vi "PathPlanner_PathFinder_ExtractPath.vi"(8 "error in (no error)":errorcluster) -> (0 "error out":errorcluster)   [LabVIEW 2019, in "PathPlanner24.lvlib"]
uses:
  PathPlanner24.lvlib
  TypeDef/PathPlannerFinderGridPosition.ctl
  PathPlanner_GridPosition_Get.vi
  PathPlanner_GridPosition_New.vi
  <vilib>/Rock Robotics/WPI/ThirdParty/JAS_Junk/TrajLib/Translation2d_Create.vi
  <vilib>/Rock Robotics/WPI/ThirdParty/JAS_Junk/TrajLib/Util_CalcDist.vi
  <vilib>/Rock Robotics/WPI/ThirdParty/JAS_Junk/TrajLib/Rotation2d_GetAngleCosSin.vi
  <vilib>/Rock Robotics/WPI/ThirdParty/JAS_Junk/TrajLib/Translation2d_GetXY.vi
  <vilib>/Rock Robotics/WPI/ThirdParty/JAS_Junk/TrajLib/Rotation2d_CreateXY.vi
  PathPlanner_PathFinder_Globals.vi
  <vilib>/Rock Robotics/WPI/ThirdParty/JAS_Junk/TrajLib/TypeDef/TRANSLATION2D.ctl
  <vilib>/Rock Robotics/WPI/ThirdParty/JAS_Junk/TrajLib/Trajectory_Library.lvlib
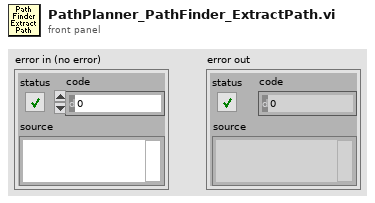
[diagram p1: front panel]
types:
  T1 = typedef "PathPlanner24.lvlib/PathPlannerFinderGridPosition.ctl" = cluster{"X":i32, "Y":i32}
  T2 = typedef "Trajectory_Library.lvlib/TRANSLATION2D.ctl" = cluster{"X":dbl, "Y":dbl}
  T3 = typedef "Trajectory_Library.lvlib/ROTATION2D.ctl" = cluster{"VALUE":dbl, "COS":dbl, "SIN":dbl}
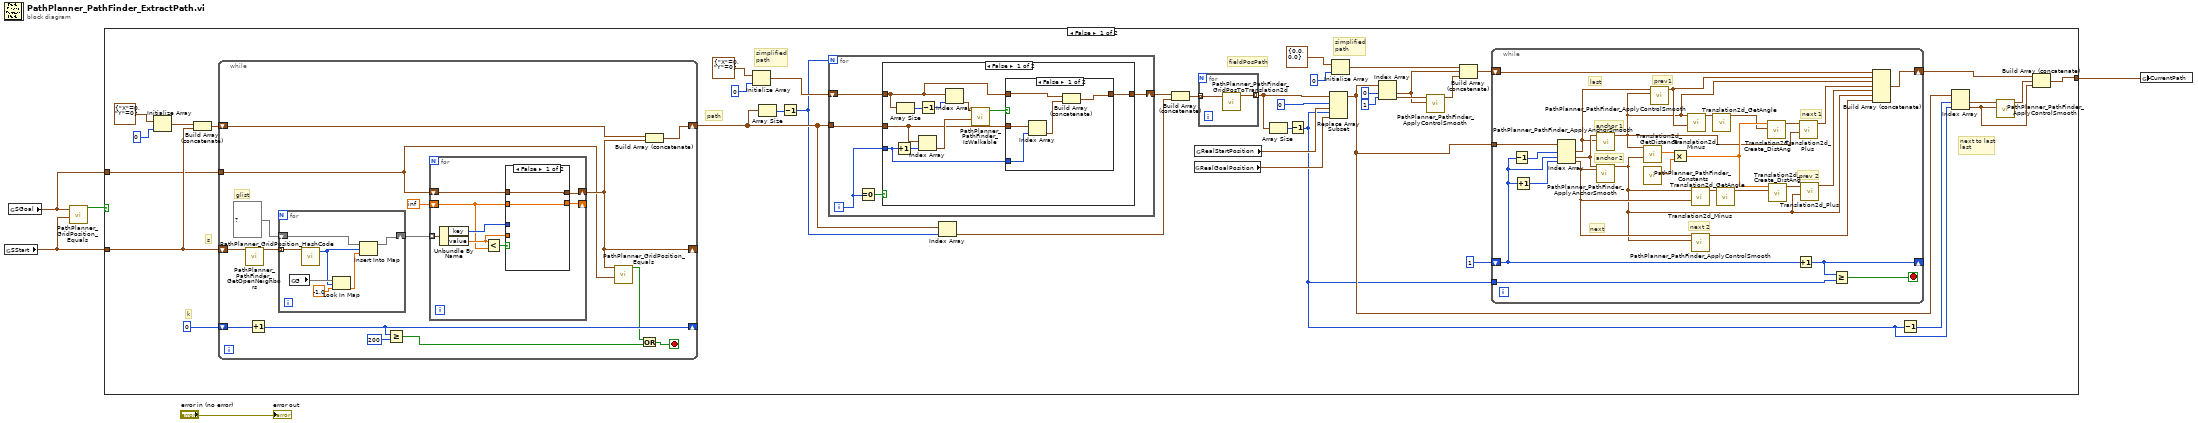
[diagram p0: block diagram]
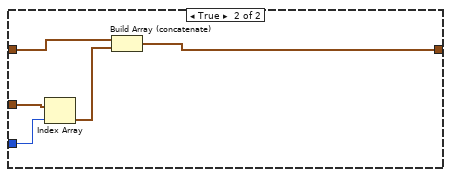
[diagram p3: hidden frame]
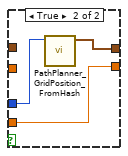
[diagram p4: hidden frame]
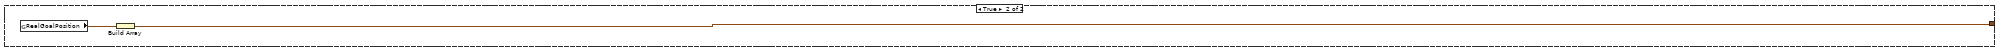
[diagram p5: hidden frame]
diagram:
  n1 = global read "PathPlanner_PathFinder_Globals.vi" "SStart"() -> (w3:T1)
  n2 = global read "PathPlanner_PathFinder_Globals.vi" "SGoal"() -> (w2:T1)
  n3 = call "PathPlanner_GridPosition_Equals.vi"("Other GridPosition"=w3, "GridPosition"=w2) -> ("Equal"=w4:bool)  [unwired: 9 in]
  n4 = case shown="False" w4 {
    tunnel: [w6 w135] -> w1
    tunnel: w3 -> [w40 _]
    tunnel: w2 -> [w39 _]
    frame False {
      # "next to last\nlast"
      # "simplified\npath"
      # "fieldPosPath"
      # "path"
      # "simplified\npath"
      # "s"
      # "k"
      n5 = Initialize Array(T1 {"X"=0, "Y"=0} ("PathPlannerFinderGridPosition"), 0 ("dimension size")) -> (w42:T1[])
      n6 = Build Array (concatenate)(w42, w40) -> (w38:T1[])
      n7 = while {
        shift-right: [w113] -> _
        shift-left: 0 -> [w114]
        tunnel: w39 -> [w101]
        shift-right: [w102] -> _
        shift-left: w40 -> [w111]
        shift-right: [w105] -> w33
        shift-left: w38 -> [w106]
        stop <- w104 stop-if-true
        # "glist"
        n8 = call "PathPlanner_PathFinder_GetOpenNeighbors.vi"("GridPosition S"=w111) -> ("Neighbors"=w110:T1[])  [unwired: 10 in]
        n9 = Increment(x=w114) -> (x+1=w113:i32)
        n10 = for {
          tunnel: w110 -> [w134] mode=indexing
          shift-right: [w128] -> w108
          shift-left: map{i32, dbl} {} ("G") -> [w131]
          n11 = global read "PathPlanner_PathFinder_Globals.vi" "G"() -> (w133:map{i32, dbl})
          n12 = call "PathPlanner_GridPosition_HashCode.vi"("GridPosition"=w134) -> ("HashCode"=w130:i32)  [unwired: 10 in]
          n13 = Look In Map(map=w133, key=w130, default value=-1.0) -> (value=w129:dbl)  [unwired: 1 out]
          n14 = Insert Into Map(map in=w131, key=w130, value=w129) -> (map out=w128:map{i32, dbl})  [unwired: 2 out]
        }
        n15 = Greater Or Equal?(x=w113, y=200) -> (x >= y?=w103:bool)
        n16 = for {
          tunnel: w108 -> [w122] mode=indexing
          shift-right: [w119] -> w102
          shift-left: w101 -> [w116]
          shift-right: [w118] -> _
          shift-left: inf -> [w115]
          n17 = Unbundle By Name(w122) -> ("key"=w120:i32, "value"=w117:dbl)
          n18 = Less?(x=w117, y=w115) -> (x < y?=w121:bool)
          n19 = case shown="False" w121 {
            tunnel: w120 -> [_ w127]
            tunnel: [w124 w126] -> w119
            tunnel: [w123 w125] -> w118
            tunnel: w117 -> [_ w125]
            tunnel: w116 -> [w124 _]
            tunnel: w115 -> [w123 _]
            frame False {
            }
            frame True {
              n20 = call "PathPlanner_GridPosition_FromHash.vi"("Hash"=w127) -> ("GridPosition"=w126:T1)  [unwired: 10 in]
            }
          }
        }
        n21 = call "PathPlanner_GridPosition_Equals.vi"("Other GridPosition"=w101, "GridPosition"=w102) -> ("Equal"=w100:bool)  [unwired: 9 in]
        n22 = Or(x=w100, y=w103) -> (x .or. y?=w104:bool)
        n23 = Build Array (concatenate)(w106, w102) -> (w105:T1[])
      }
      n24 = Initialize Array(T1 {"X"=0, "Y"=0} ("PathPlannerFinderGridPosition"), 0 ("dimension size")) -> (w35:T1[])
      n25 = Array Size(array=w33) -> (size(s)=w34:i32)
      n26 = Decrement(x=w34) -> (x-1=w32:i32)
      n27 = for {
        N: w32 -> [_]
        shift-right: [w76] -> w31
        shift-left: w35 -> [w77]
        tunnel: w33 -> [w75]
        i -> [w74]
        n28 = Equal To 0?(x=w74) -> (x = 0?=w78:bool)
        n29 = case shown="False" w78 {
          tunnel: w77 -> [w82 w99]
          tunnel: [w81 w98] -> w76
          tunnel: w75 -> [w80 w97]
          tunnel: w74 -> [w79 w96]
          frame False {
            n30 = Increment(x=w79) -> (x+1=w88:i32)
            n31 = Array Size(array=w82) -> (size(s)=w86:i32)
            n32 = Index Array(array=w80, index=w88) -> (element=w87:T1)
            n33 = Decrement(x=w86) -> (x-1=w85:i32)
            n34 = Index Array(array=w82, index=w85) -> (element=w84:T1)
            n35 = call "PathPlanner_PathFinder_IsWalkable.vi"("S2"=w87, "S1"=w84) -> ("IsWalkable"=w83:bool)  [unwired: 9 in]
            n36 = case shown="False" w83 {
              tunnel: w82 -> [w93 w94]
              tunnel: [w92 w94] -> w81
              tunnel: w80 -> [w91 _]
              tunnel: w79 -> [w90 _]
              frame False {
                n37 = Index Array(array=w91, index=w90) -> (element=w89:T1)
                n38 = Build Array (concatenate)(w93, w89) -> (w92:T1[])
              }
              frame True {
              }
            }
          }
          frame True {
            n39 = Index Array(array=w97, index=w96) -> (element=w95:T1)
            n40 = Build Array (concatenate)(w99, w95) -> (w98:T1[])
          }
        }
      }
      n41 = Index Array(array=w33, index=w32) -> (element=w30:T1)
      n42 = Build Array (concatenate)(w31, w30) -> (w29:T1[])
      n43 = global read "PathPlanner_PathFinder_Globals.vi" "RealGoalPosition"() -> (w24:T2)
      n44 = global read "PathPlanner_PathFinder_Globals.vi" "RealStartPosition"() -> (w27:T2)
      n45 = for {
        tunnel: w29 -> [w73] mode=indexing
        tunnel: [w72] -> w25 mode=indexing
        n46 = call "PathPlanner_PathFinder_GridPosToTranslation2d.vi"("GridPosition"=w73) -> ("RealGridPos"=w72:T2)  [unwired: 10 in]
      }
      n47 = Array Size(array=w25) -> (size(s)=w26:i32)
      n48 = Decrement(x=w26) -> (x-1=w11:i32)
      n49 = Replace Array Subset(array=w25, new element #1=w27, index #1=0 ("index"), new element #2=w24, index #2=w11) -> (w13:T2[])
      n50 = Initialize Array(T2 {"X"=0.0, "Y"=0.0} ("TRANSLATION2D"), 0 ("dimension size")) -> (w20:T2[])
      n51 = Index Array(array=w13, index #1=0 ("index"), index #2=1 ("index")) -> (element #1=w15:T2, element #2=w16:T2)
      n52 = call "PathPlanner_PathFinder_ApplyControlSmooth.vi"("Current"=w15, "Other"=w16) -> ("Smoothed"=w14:T2)  [unwired: 9 in]
      n53 = Build Array (concatenate)(w20, w15, w14) -> (w18:T2[])
      n54 = while {
        shift-right: [w45] -> w10
        shift-left: w18 -> [w52]
        shift-right: [w71] -> _
        shift-left: 1 -> [w66]
        tunnel: w11 -> [w70]
        tunnel: w13 -> [w68]
        stop <- w69 stop-if-true
        # "prev 2"
        # "last"
        # "next"
        # "next 1"
        # "next 2"
        # "prev1"
        # "anchor 2"
        # "anchor 1"
        n55 = Decrement(x=w66) -> (x-1=w67:i32)
        n56 = Increment(x=w66) -> (x+1=w65:i32)
        n57 = Index Array(array=w68, index #1=w67, index #2=w66, index #3=w65) -> (element #1=w59:T2, element #2=w64:T2, element #3=w54:T2)
        n58 = call "PathPlanner_PathFinder_ApplyAnchorSmooth.vi"("Current"=w54, "Other"=w64) -> ("Smoothed"=w47:T2)  [unwired: 9 in]
        n59 = call "PathPlanner_PathFinder_ApplyAnchorSmooth.vi"("Current"=w59, "Other"=w64) -> ("Smoothed"=w50:T2)  [unwired: 9 in]
        n60 = call <vilib>:"Translation2d_GetDistance.vi"("other Translation"=w47, "In Translation"=w50) -> ("Distance"=w63:dbl)  [unwired: 9 in]
        n61 = call "PathPlanner_PathFinder_Constants.vi"() -> ("SMOOTHING_CONTROL_PCT"=w62:dbl)  [unwired: 9 in, 2 out]
        n62 = call "PathPlanner_PathFinder_ApplyControlSmooth.vi"("Current"=w50, "Other"=w59) -> ("Smoothed"=w51:T2)  [unwired: 9 in]
        n63 = Multiply(x=w63, y=w62) -> (x*y=w61:dbl)
        n64 = call <vilib>:"Translation2d_Minus.vi"("other Translation"=w51, "In Translation"=w50) -> ("Out Translation"=w60:T2)  [unwired: 9 in]
        n65 = call <vilib>:"Translation2d_Minus.vi"("other Translation"=w54, "In Translation"=w47) -> ("Out Translation"=w57:T2)  [unwired: 9 in]
        n66 = call "PathPlanner_PathFinder_ApplyControlSmooth.vi"("Current"=w47, "Other"=w54) -> ("Smoothed"=w46:T2)  [unwired: 9 in]
        n67 = call <vilib>:"Translation2d_GetAngle.vi"("In Translation"=w60) -> ("Angle_Rotation2d"=w58:T3)  [unwired: 10 in]
        n68 = call <vilib>:"Translation2d_GetAngle.vi"("In Translation"=w57) -> ("Angle_Rotation2d"=w56:T3)  [unwired: 10 in]
        n69 = call <vilib>:"Translation2d_Create_DistAng.vi"("Angle"=w58, "Dist"=w61) -> ("TRANSLATION"=w55:T2)  [unwired: 9 in]
        n70 = call <vilib>:"Translation2d_Create_DistAng.vi"("Angle"=w56, "Dist"=w61) -> ("TRANSLATION"=w53:T2)  [unwired: 9 in]
        n71 = Increment(x=w66) -> (x+1=w71:i32)
        n72 = call <vilib>:"Translation2d_Plus.vi"("other Translation"=w50, "In Translation"=w55) -> ("Out Translation"=w49:T2)  [unwired: 9 in]
        n73 = call <vilib>:"Translation2d_Plus.vi"("other Translation"=w47, "In Translation"=w53) -> ("Out Translation"=w48:T2)  [unwired: 9 in]
        n74 = Greater Or Equal?(x=w71, y=w70) -> (x >= y?=w69:bool)
        n75 = Build Array (concatenate)(w52, w51, w50, w49, w48, w47, w46) -> (w45:T2[])
      }
      n76 = Decrement(x=w11) -> (x-1=w12:i32)
      n77 = Index Array(array=w13, index #1=w12, index #2=w11) -> (element #1=w9:T2, element #2=w7:T2)
      n78 = call "PathPlanner_PathFinder_ApplyControlSmooth.vi"("Current"=w7, "Other"=w9) -> ("Smoothed"=w8:T2)  [unwired: 9 in]
      n79 = Build Array (concatenate)(w10, w8, w7) -> (w6:T2[])
    }
    frame True {
      n80 = global read "PathPlanner_PathFinder_Globals.vi" "RealGoalPosition"() -> (w136:T2)
      n81 = Build Array(w136) -> (w135:T2[])
    }
  }
  n82 = global write "PathPlanner_PathFinder_Globals.vi" "CurrentPath"(w1) -> ()
  "error out" <- "error in (no error)"
